vi "2sComp to Decimal.vi"(10 "size in bit":i16=2057, 11 "word in":u16=2057 format="%.0b") -> (3 "decimal out":i16)   [LabVIEW 2020, in "dt_encodeDecode.lvlib"]
uses:
  dt_encodeDecode.lvlib
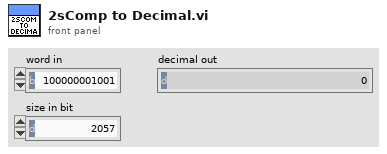
[diagram p1: front panel]
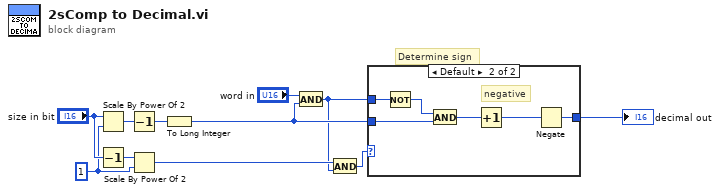
[diagram p0: block diagram]
diagram:
  w6 = u32 1 ("x")
  # "Determine sign"
  n1 = Scale By Power Of 2(n="size in bit", x=w6) -> (x*2^n=w5:u32)
  n2 = Decrement(x="size in bit") -> (x-1=w8:i16)
  n3 = Decrement(x=w5) -> (x-1=w3:u32)
  n4 = Scale By Power Of 2(n=w8, x=w6) -> (x*2^n=w4:u32)
  n5 = To Long Integer(number=w3) -> (32bit integer=w2:i32)
  n6 = And(x="word in", y=w2) -> (x .and. y?=w1:i32)
  n7 = And(x=w4, y=w1) -> (x .and. y?=w10:u32)
  n8 = case shown="Default" w10 {
    tunnel: [w12 w14] -> w9
    tunnel: w1 -> [w12 w18]
    tunnel: w2 -> [_ w15]
    frame 0 {
      # "positive"
    }
    frame Default {
      # "negative"
      n9 = Not(x=w18) -> (.not. x?=w17:i32)
      n10 = And(x=w17, y=w15) -> (x .and. y?=w16:i32)
      n11 = Increment(x=w16) -> (x+1=w13:i32)
      n12 = Negate(x=w13) -> (-x=w14:i32)
    }
  }
  "decimal out" <- w9
